vi "write read test.vi"(10 "readOut":u8[](array[numeric])=[0, 0, 0, 0], 11 "idx":u32) -> (2 "readOut out":u8[](array[numeric]), 3 "function return":bool)   [LabVIEW 2018, in "Dll1_x64_191014_0.lvlib"]
doc: "__declspec(dllexport) bool write_read_test(unsigned int idx, unsigned char readOut[4]);"
uses:
  <userlib>/Dll1_x64_191014_0/Dll1_x64_191014_0.lvlib
  <userlib>/Dll1_x64_191014_0/Dll1.dll
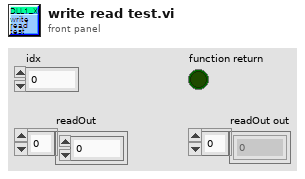
[diagram p1: front panel]
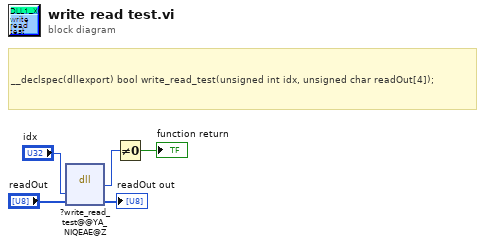
[diagram p0: block diagram]
diagram:
  # "__declspec(dllexport) bool write_read_test(unsigned int idx, unsigned char readOut[4]);"
  n1 = dll-call lib="C:/Program Files/National Instruments/LabVIEW 2018/user.lib/Dll1_x64_191014_0/Dll1.*" fn="?write_read_test@@YA_NIQEAE@Z"("idx"="idx", "readOut"="readOut") -> (w4:u8, "readOut"=→"readOut out":u8[])  [unwired: 4 in, 2 out]
  n2 = Not Equal To 0?(x=w4) -> (x != 0?=→"function return":bool)
